vi "Get Number of Columns in Table.vi"(4 "Table in":dbl[][](array[numeric])) -> (1 "# Columns":i32)   [LabVIEW 2018, in "Potentiostat Galvanostat.lvclass"]
uses:
  Potentiostat Galvanostat.lvclass
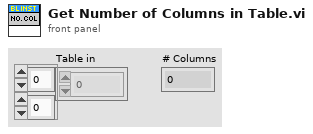
[diagram p1: front panel]
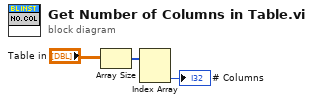
[diagram p0: block diagram]
diagram:
  n1 = Array Size(array="Table in") -> (size(s)=w2:i32[])
  n2 = Index Array(array=w2) -> (element #2=→"# Columns":i32)  [unwired: 2 in, 1 out]
